vi "dfd_Convert Coefficients String to Filter.vi"(8 "error in (no error)":errorcluster, 10 "xml string in":string, 11 "filter":T1={"mSRate_Fs"=1.0, "mSRate_Version"="1.0", "mSRate_Comments"="", "mSRate_OrgCoef"={"type"=enum."Undefined", "gain"=1.0, "coef a (k)"=[], "coef b (v)"=[]}, "mSRate_CurCoef"={"type"=enum."Undefined", "gain"=1.0, "coef a (k)"=[], "coef b (v)"=[]}, "mSRate_Quantized?"=FALSE, "mSRate_QCoef"={"type"=enum."Undefined", "gain"=1.0, "coef a (k)"=[], "coef b (v)"=[]}, "mSRate_QSettings"=[], "mSRate_Order"=0, "mSRate_Scaling"={"mSRate_ScaleByPowerOf2?"=FALSE, "mSRate_ScaleType"=enum."No Norm"}} {"mSRate_QSettings"."source" items=["Coef a/k"=0, "Coef b/v"=7, "Input"=1, "Output"=2, "Multiplicand"=3, "Product"=4, "Sum"=5, "Delay"=6, "Gain"=8]}) -> (0 "error out":errorcluster, 3 "filter out":T1={"mSRate_Fs"=1.0, "mSRate_Version"="1.0", "mSRate_Comments"="", "mSRate_OrgCoef"={"type"=enum."Undefined", "gain"=1.0, "coef a (k)"=[], "coef b (v)"=[]}, "mSRate_CurCoef"={"type"=enum."Undefined", "gain"=1.0, "coef a (k)"=[], "coef b (v)"=[]}, "mSRate_Quantized?"=FALSE, "mSRate_QCoef"={"type"=enum."Undefined", "gain"=1.0, "coef a (k)"=[], "coef b (v)"=[]}, "mSRate_QSettings"=[], "mSRate_Order"=0, "mSRate_Scaling"={"mSRate_ScaleByPowerOf2?"=FALSE, "mSRate_ScaleType"=enum."No Norm"}} {"mSRate_QSettings"."source" items=["Coef a/k"=0, "Coef b/v"=7, "Input"=1, "Output"=2, "Multiplicand"=3, "Product"=4, "Sum"=5, "Delay"=6, "Gain"=8]})   [LabVIEW 2017, in "NI_DigFilter_Process.lvlib"]
uses:
  <vilib>/addons/Digital Filter Design/NI_DigFilter_Process.lvlib
  <vilib>/addons/Digital Filter Design/_Objects.llb/DFD Filter Obj.ctl
  <vilib>/addons/Digital Filter Design/_Objects.llb/DFD Filter Coef.ctl
  <vilib>/addons/Digital Filter Design/_Objects.llb/DFD Filter Structure Type Selector.ctl
  <vilib>/addons/Digital Filter Design/_Objects.llb/dfd_Internal Quantization Settings.ctl
  <vilib>/addons/Digital Filter Design/_Objects.llb/dfd_Internal Quantization Srcs.ctl
  <vilib>/addons/Digital Filter Design/_Objects.llb/DFD Coef Norm Type.ctl
  <vilib>/addons/Digital Filter Design/NI_DigFilterLicensed.lvlib
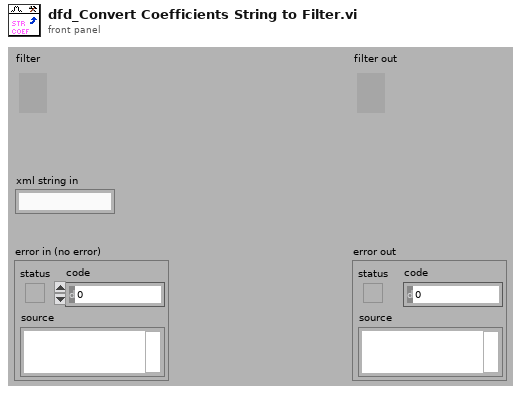
[diagram p1: front panel]
types:
  T1 = typedef "NI_DigFilterLicensed.lvlib/DFD Filter Obj.ctl" = cluster{"mSRate_Fs":dbl, "mSRate_Version":string, "mSRate_Comments":string, "mSRate_OrgCoef":T2, "mSRate_CurCoef":T2, "mSRate_Quantized?":bool, "mSRate_QCoef":T2, "mSRate_QSettings":T4[], "mSRate_Order":i32, "mSRate_Scaling":cluster{"mSRate_ScaleByPowerOf2?":bool, "mSRate_ScaleType":T6}}
  T2 = typedef "NI_DigFilterLicensed.lvlib/DFD Filter Coef.ctl" = cluster{"type":T3, "gain":dbl, "coef a (k)":dbl[], "coef b (v)":dbl[]}
  T3 = typedef "NI_DigFilterLicensed.lvlib/DFD Filter Structure Type Selector.ctl" = enum16{"Undefined", "FIR Direct Form", "FIR Direct Form Transposed", "FIR Symmetric", "FIR Antisymmetric", "IIR Direct Form I", "IIR Direct Form I Transposed", "IIR Direct Form II", "IIR Direct Form II Transposed", "IIR Cascaded Second Order Sections Form I", "IIR Cascaded Second Order Sections Form I Transposed", "IIR Cascaded Second Order Sections Form II", "IIR Cascaded Second Order Sections Form II Transposed", "Lattice Allpass (basic sections)", "Lattice Allpass (one multiplier sections)", "Lattice Allpass (normalized sections)", "Lattice AR (basic sections)", "Lattice AR (one multiplier sections)", "Lattice AR (normalized sections)", "Lattice MA (minimum phase)", "Lattice MA (maximum phase)", "Lattice ARMA (basic sections)", "Lattice ARMA (one multiplier sections)", "Lattice ARMA (normalized sections)"}
  T4 = typedef "NI_DigFilterLicensed.lvlib/dfd_Internal Quantization Settings.ctl" = cluster{"source":T5, "wl":i16, "iwl":i16, "overflow mode":enum16{"Saturation", "Wrap"}, "rounding mode":enum16{"Nearest", "Truncation"}, "signed?":bool}
  T5 = typedef "NI_DigFilterLicensed.lvlib/dfd_Internal Quantization Srcs.ctl" = u16
  T6 = typedef "NI_DigFilterLicensed.lvlib/DFD Coef Norm Type.ctl" = enum16{"No Norm", "Time Domain 1-Norm", "Time Domain 2-Norm", "Time Domain Inf-Norm"}
  T7 = cluster{"type":T3, "numeric array":dbl[], "numeric array":dbl[], "value":dbl}
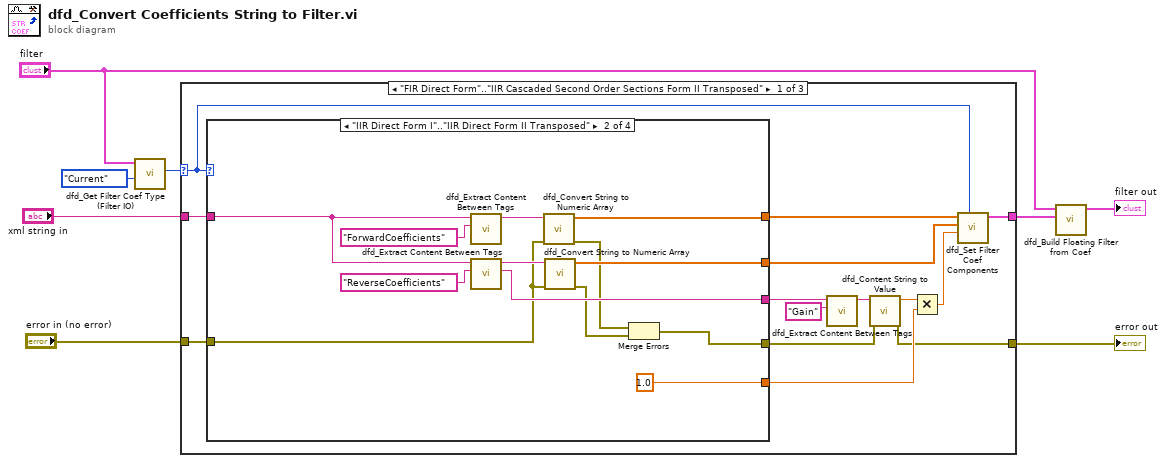
[diagram p0: block diagram]
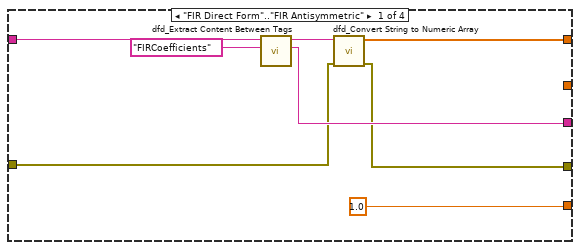
[diagram p2: hidden frame]
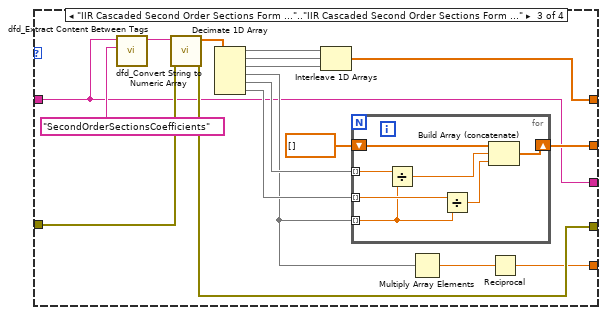
[diagram p3: hidden frame]
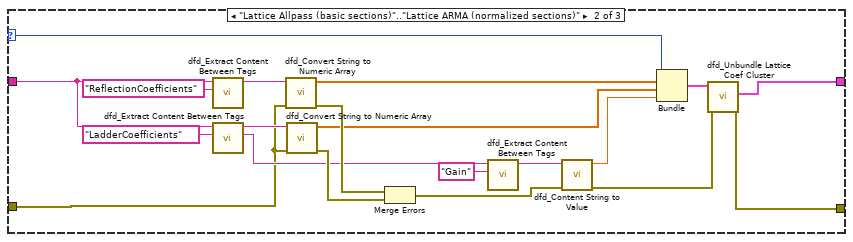
[diagram p5: hidden frame]
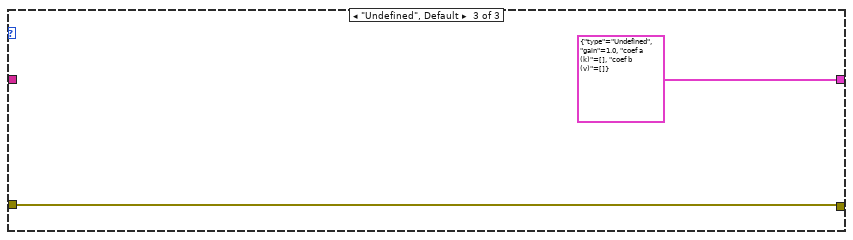
[diagram p6: hidden frame]
diagram:
  n1 = call <vilib>:"dfd_Get Filter Coef Type (Filter IO).vi"("coef source"=enum16{"Original", "Current", "Quantized"}."Current", "filter in"="filter") -> ("type"=w2:T3)  [unwired: 1 in, 8 out]
  n2 = case shown="\"FIR Direct Form\"..\"IIR Cascaded Second Order Sections Form II Transposed\"" w2 {
    selector: w2 -> [w14 w75 _]
    tunnel: "xml string in" -> [w22 w79 _]
    tunnel: [w9 w69 w88] -> w7
    tunnel: "error in (no error)" -> [w18 w71 w88]
    tunnel: [w16 w70 T2 {"type"=enum."Undefined", "gain"=1.0, "coef a (k)"=[], "coef b (v)"=[]} ("filter coef")] -> w5
    frame "FIR Direct Form".."IIR Cascaded Second Order Sections Form II Transposed" {
      n3 = case shown="\"IIR Direct Form I\"..\"IIR Direct Form II Transposed\"" w14 {
        tunnel: [w28 w37 w46 _] -> w21
        tunnel: w22 -> [w30 w36 w46 _]
        tunnel: w18 -> [w26 w31 w56 _]
        tunnel: [w25 w33 w55 _] -> w10
        tunnel: [w24 w40 w50 _] -> w17
        tunnel: [_ w38 w60 _] -> w15
        tunnel: [1.0 1.0 ("x") w44 _] -> w11
        frame "FIR Direct Form".."FIR Antisymmetric" {
          n4 = call <vilib>:"dfd_Extract Content Between Tags.vi"("element"="FIRCoefficients", "xml string with tag"=w30) -> ("remaining string"=w28:string, "content"=w27:string)  [unwired: 8 out]
          n5 = call <vilib>:"dfd_Convert String to Numeric Array.vi"("error in"=w26, "string"=w27) -> ("error out"=w25:errorcluster, "numeric array"=w24:dbl[])  [unwired: 8 out]
        }
        frame "IIR Direct Form I".."IIR Direct Form II Transposed" {
          n6 = call <vilib>:"dfd_Extract Content Between Tags.vi"("element"="ForwardCoefficients", "xml string with tag"=w36) -> ("content"=w42:string)  [unwired: 9 out]
          n7 = call <vilib>:"dfd_Extract Content Between Tags.vi"("element"="ReverseCoefficients", "xml string with tag"=w36) -> ("remaining string"=w37:string, "content"=w39:string)  [unwired: 8 out]
          n8 = call <vilib>:"dfd_Convert String to Numeric Array.vi"("error in"=w31, "string"=w42) -> ("error out"=w35:errorcluster, "numeric array"=w40:dbl[])  [unwired: 8 out]
          n9 = call <vilib>:"dfd_Convert String to Numeric Array.vi"("error in"=w31, "string"=w39) -> ("error out"=w34:errorcluster, "numeric array"=w38:dbl[])  [unwired: 8 out]
          n10 = Merge Errors(w35, w34) -> (w33:errorcluster)
        }
        frame "IIR Cascaded Second Order Sections Form I".."IIR Cascaded Second Order Sections Form II Transposed" {
          n11 = call <vilib>:"dfd_Extract Content Between Tags.vi"("element"="SecondOrderSectionsCoefficients", "xml string with tag"=w46) -> ("content"=w59:string)  [unwired: 9 out]
          n12 = call <vilib>:"dfd_Convert String to Numeric Array.vi"("error in"=w56, "string"=w59) -> ("error out"=w55:errorcluster, "numeric array"=w54:dbl[])  [unwired: 8 out]
          n13 = Decimate 1D Array(w54) -> (w53:dbl[], w52:dbl[], w51:dbl[], w47:dbl[], w49:dbl[], w48:dbl[])
          n14 = Interleave 1D Arrays(w53, w52, w51) -> (w50:dbl[])
          n15 = for {
            shift-right: [w67] -> w60
            shift-left: dbl[] [] -> [w66]
            tunnel: w47 -> [w63] mode=indexing
            tunnel: w49 -> [w65] mode=indexing
            tunnel: w48 -> [w64] mode=indexing
            n16 = Divide(x=w65, y=w63) -> (x/y=w62:dbl)
            n17 = Divide(x=w64, y=w63) -> (x/y=w61:dbl)
            n18 = Build Array (concatenate)(w66, w62, w61) -> (w67:dbl[])
          }
          n19 = Multiply Array Elements(1:w47) -> (0:w45:dbl)
          n20 = Reciprocal(x=w45) -> (1/x=w44:dbl)
        }
        frame Default {
        }
      }
      n21 = call <vilib>:"dfd_Extract Content Between Tags.vi"("element"="Gain", "xml string with tag"=w21) -> ("content"=w20:string)  [unwired: 9 out]
      n22 = call <vilib>:"dfd_Content String to Value.vi"("error in (no error)"=w10, "string"=w20) -> ("error out"=w9:errorcluster, "value"=w13:dbl)  [unwired: 8 out]
      n23 = Multiply(x=w13, y=w11) -> (x*y=w12:dbl)
      n24 = call <vilib>:"dfd_Set Filter Coef Components.vi"("type"=w14, "gain"=w12, "coef a (k)"=w15, "coef b (v)"=w17) -> ("filter coef"=w16:T2)  [unwired: 1 in, 6 out]
    }
    frame "Lattice Allpass (basic sections)".."Lattice ARMA (normalized sections)" {
      n25 = call <vilib>:"dfd_Extract Content Between Tags.vi"("element"="ReflectionCoefficients", "xml string with tag"=w79) -> ("content"=w84:string)  [unwired: 9 out]
      n26 = call <vilib>:"dfd_Extract Content Between Tags.vi"("element"="LadderCoefficients", "xml string with tag"=w79) -> ("remaining string"=w78:string, "content"=w82:string)  [unwired: 8 out]
      n27 = call <vilib>:"dfd_Convert String to Numeric Array.vi"("error in"=w71, "string"=w84) -> ("error out"=w81:errorcluster, "numeric array"=w74:dbl[])  [unwired: 8 out]
      n28 = call <vilib>:"dfd_Convert String to Numeric Array.vi"("error in"=w71, "string"=w82) -> ("error out"=w80:errorcluster, "numeric array"=w73:dbl[])  [unwired: 8 out]
      n29 = Merge Errors(w81, w80) -> (w77:errorcluster)
      n30 = call <vilib>:"dfd_Extract Content Between Tags.vi"("element"="Gain", "xml string with tag"=w78) -> ("content"=w87:string)  [unwired: 9 out]
      n31 = call <vilib>:"dfd_Content String to Value.vi"("error in (no error)"=w77, "string"=w87) -> ("error out"=w68:errorcluster, "value"=w72:dbl)  [unwired: 8 out]
      n32 = Bundle("type"=w75, "numeric array"=w74, "numeric array"=w73, "value"=w72) -> (w76:T7)  [unwired: 1 out]
      n33 = call <vilib>:"dfd_Unbundle Lattice Coef Cluster.vi"("error in (no error)"=w68, "Lattice coef"=w76) -> ("error out"=w69:errorcluster, "filter coef out"=w70:T2)  [unwired: 8 out]
    }
    frame "Undefined", Default {
    }
  }
  "error out" <- w7
  n34 = call <vilib>:"dfd_Build Floating Filter from Coef.vi"("filter coef"=w5, "filter in"="filter") -> ("filter out"=→"filter out":T1)  [unwired: 2 in, 7 out]
